vi "Draw Crosshair.vi"(6 "Length":i32, 7 "Thickness":i32, 8 "Color":u32(colorbox)=16711680, 9 "Y":dbl, 10 "X":dbl, 11 "Image in":T1) -> (3 "Image out":T1)   [LabVIEW 2015]
uses:
  <vilib>/vision/Image Controls.llb/IMAQ Image.ctl
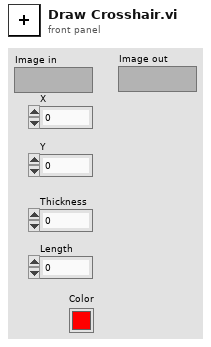
[diagram p1: front panel]
types:
  T1 = typedef "IMAQ Image.ctl" = refnum<image>
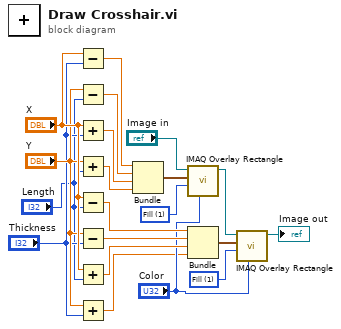
[diagram p0: block diagram]
diagram:
  w13 = u32 1 items=["Frame", "Fill", "Highlight"] ("Drawing Mode (Frame)")
  w7 = u32 1 items=["Frame", "Fill", "Highlight"] ("Drawing Mode (Frame)")
  n1 = Subtract(x="X", y="Thickness") -> (x-y=w9:dbl)
  n2 = Subtract(x="Y", y="Length") -> (x-y=w10:dbl)
  n3 = Add(x="X", y="Thickness") -> (x+y=w11:dbl)
  n4 = Add(x="Y", y="Length") -> (x+y=w12:dbl)
  n5 = Subtract(x="X", y="Length") -> (x-y=w17:dbl)
  n6 = Subtract(x="Y", y="Thickness") -> (x-y=w18:dbl)
  n7 = Add(x="X", y="Length") -> (x+y=w19:dbl)
  n8 = Add(x="Y", y="Thickness") -> (x+y=w4:dbl)
  n9 = Bundle(w9, w10, w11, w12) -> (w8:cluster{dbl, dbl, dbl, dbl})  [unwired: 1 in]
  n10 = call "IMAQ Overlay Rectangle"("Color"="Color", "Drawing Mode (Frame)"=w7, "Rectangle"=w8, "Image"="Image in") -> ("Image Out"=w14:T1)  [unwired: 6 in, 1 out]
  n11 = Bundle(w17, w18, w19, w4) -> (w16:cluster{dbl, dbl, dbl, dbl})  [unwired: 1 in]
  n12 = call "IMAQ Overlay Rectangle"("Color"="Color", "Drawing Mode (Frame)"=w13, "Rectangle"=w16, "Image"=w14) -> ("Image Out"=→"Image out":T1)  [unwired: 6 in, 1 out]
